vi "SetVarVal_Array.vi"(8 "error in (no error)":errorcluster, 9 "varValue":dbl[](array[numeric]), 10 "varName":string, 11 "muExpr in":refnum<class "mupExpr.lvclass">) -> (0 "error out":errorcluster, 3 "muExpr out":refnum<class "mupExpr.lvclass">)   [LabVIEW 2015, in "mupExpr.lvclass"]
uses:
  mupExpr.lvclass
  mupExpr.lvclass/mupExpr.ctl
  mupLib/mupLib.lvlib
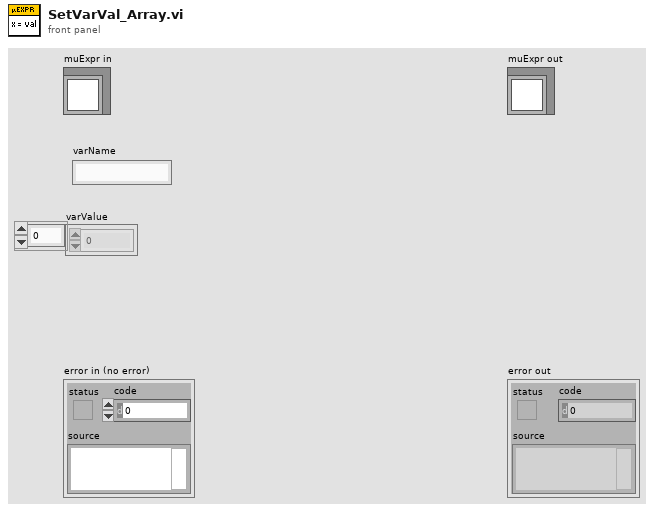
[diagram p1: front panel]
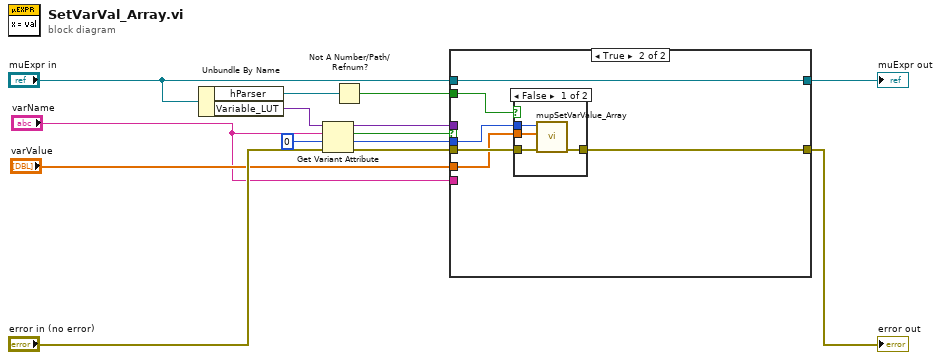
[diagram p0: block diagram]
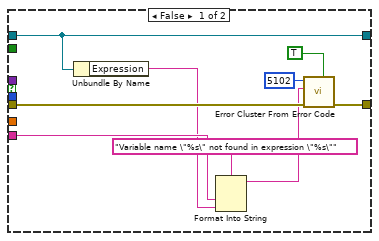
[diagram p2: hidden frame]
diagram:
  n1 = Unbundle By Name("muExpr in") -> ("hParser"=w2:refnum<data-value>, "Variable_LUT"=w8:variant)
  n2 = Get Variant Attribute(Variant=w8, name="varName", default value (empty Variant)=u64 0 ("pd"), error in="error in (no error)") -> (duplicate Variant=w3:variant, found=w4:bool, value=w5:u64, error out=w7:errorcluster)
  n3 = Not A Number/Path/Refnum?(number/path/refnum=w2) -> (NaN/Path/Refnum?=w1:bool)
  n4 = case shown="True" w4 {
    tunnel: w7 -> [w23 w28]
    tunnel: "varValue" -> [_ w26]
    tunnel: w5 -> [_ w25]
    tunnel: [w21 w27] -> w13
    tunnel: "varName" -> [w20 _]
    tunnel: "muExpr in" -> [w22 w29]
    tunnel: w3 -> [_ _]
    tunnel: [w22 w29] -> w11
    tunnel: w1 -> [_ w24]
    frame False {
      n5 = Unbundle By Name(w22) -> ("Expression"=w17:string)
      n6 = Format Into String(format string="Variable name \"%s\" not found in expression \"%s\"", w20, w17) -> (resulting string=w16:string)  [unwired: 2 in, 1 out]
      n7 = call <vilib>:"Error Cluster From Error Code.vi"("is warning? (False)"=TRUE, "error in (no error)"=w23, "error message (\"\")"=w16, "error code (0)"=5102) -> ("error out"=w21:errorcluster)  [unwired: 5 in]
    }
    frame True {
      n8 = case shown="False" w24 {
        tunnel: w28 -> [w33 w34]
        tunnel: [w32 w34] -> w27
        tunnel: w26 -> [w31 _]
        tunnel: w25 -> [w30 _]
        frame False {
          n9 = call "mupSetVarValue_Array.vi"("error in (no error)"=w33, "varValue"=w31, "varPtr in"=w30) -> ("error out"=w32:errorcluster)  [unwired: 7 in, 1 out]
        }
        frame True {
        }
      }
    }
  }
  "error out" <- w13
  "muExpr out" <- w11
